vi "Write Multiple Registers.vi"(8 "error in":errorcluster, 9 "register values":u16[](array[numeric]), 10 "starting address":u16, 11 "device data model in":refnum<class "Standard Data Model.lvclass">) -> (0 "error out":errorcluster, 3 "device data model out":refnum<class "Standard Data Model.lvclass">)   [LabVIEW 2013, in "Modbus Library - Advance.lvlib" / "Standard Data Model.lvclass"]
doc: "Writes the values of multiple register values in series, starting at address M."
uses:
  Standard Data Model.lvclass
  Standard Data Model.lvclass/Standard Data Model.ctl
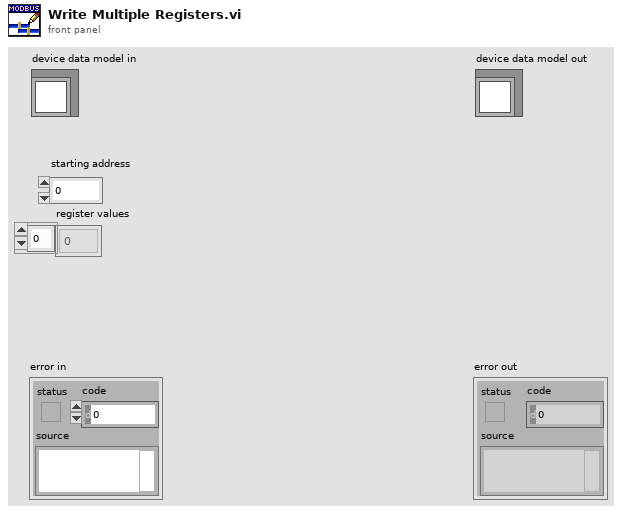
[diagram p1: front panel]
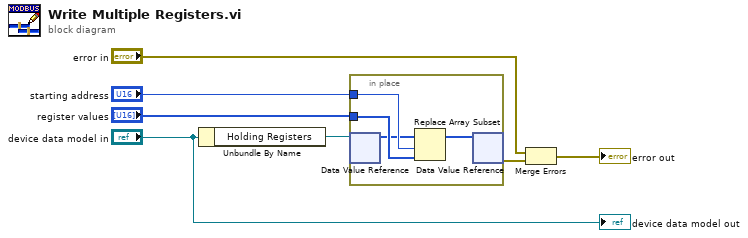
[diagram p0: block diagram]
diagram:
  n1 = Unbundle By Name("device data model in") -> ("Holding Registers"=w4:refnum<data-value>)
  n2 = in-place {
    in-place-border: "register values" -> [w11]
    in-place-border: "starting address" -> [w10]
    n3 = in-place-dvr #1(w4) -> (w9:u16[])  [unwired: 1 out]
    n4 = Replace Array Subset(array=w9, new element=w11, index=w10) -> (w8:u16[])
    n5 = in-place-dvr #1(w8) -> (w5:errorcluster)  [unwired: 1 out]
  }
  n6 = Merge Errors("error in", w5) -> (→"error out":errorcluster)
  "device data model out" <- "device data model in"
